vi "init_double_check_moving.vi"(8 "error in (no error)":errorcluster, 11 "MotorSystem in":refnum<class "MotorSystem.lvclass">) -> (0 "error out":errorcluster, 3 "MotorSystem out":refnum<class "MotorSystem.lvclass">)   [LabVIEW 2016, in "MotionControl_UFO_3DOF.lvlib" / "MotorSystem.lvclass"]
uses:
  <userlib>/MotionControl_UFO_3DOF/MotorSystem/MotorSystem.lvclass
  <userlib>/MotionControl_UFO_3DOF/MotorSystem/MotorSystem.lvclass/MotorSystem.ctl
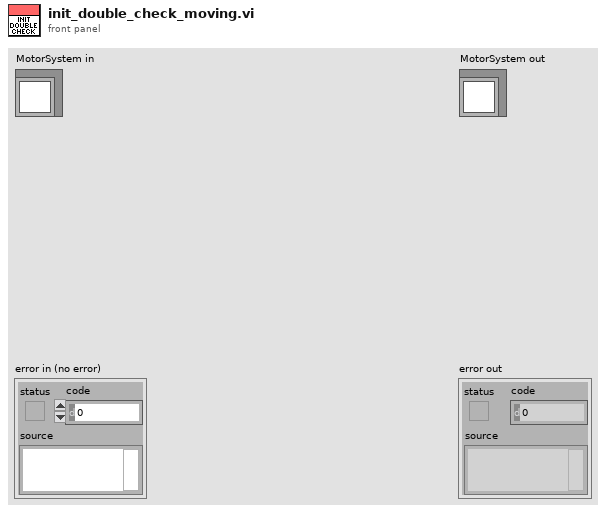
[diagram p1: front panel]
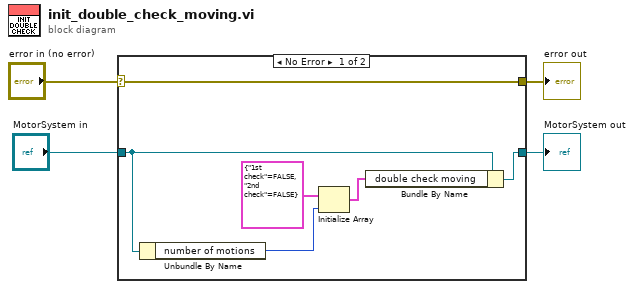
[diagram p0: block diagram]
diagram:
  n1 = case shown="No Error" "error in (no error)" {
    selector: "error in (no error)" -> [w10 w11]
    tunnel: [w10 w11] -> w3
    tunnel: [w9 w12] -> w1
    tunnel: "MotorSystem in" -> [w7 w12]
    frame No Error {
      n2 = Unbundle By Name(w7) -> ("number of motions"=w6:i32)
      n3 = Initialize Array(cluster{"1st check":bool, "2nd check":bool} {"1st check"=FALSE, "2nd check"=FALSE}, w6) -> (w5:cluster{"1st check":bool, "2nd check":bool}[])
      n4 = Bundle By Name(cluster=w7, "double check moving"=w5) -> (w9:refnum<class "MotorSystem.lvclass">)
    }
    frame Error {
    }
  }
  "error out" <- w3
  "MotorSystem out" <- w1
